vi "实验配置信息读取和写入.vi"(1 "读取写入":bool, 3 "输入簇":T1) -> (9 "输出簇":T1)   [LabVIEW 2010]
uses:
  <vilib>/Utility/config.llb/Read Key (String).vi
  <vilib>/Utility/config.llb/Write Key (String).vi
  <vilib>/Utility/config.llb/NI_LVConfig.lvlib
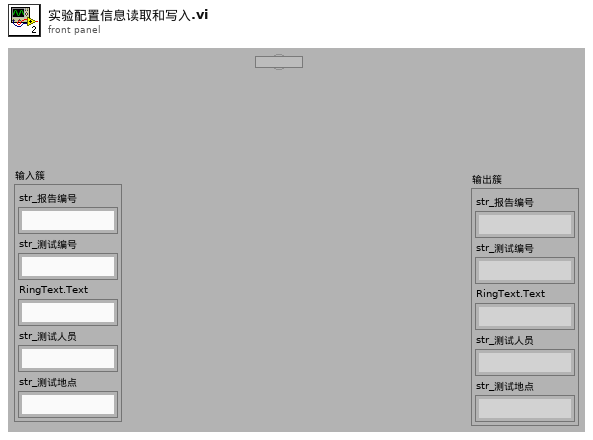
[diagram p1: front panel]
types:
  T1 = cluster{"str_报告编号":string, "str_测试编号":string, "RingText.Text":string, "str_测试人员":string, "str_测试地点":string}
  T2 = typedef "NI_LVConfig.lvlib/Config Data RefNum.ctl" = refnum<k1>
  T3 = cluster{"value":string, "value":string, "value":string, "value":string, "value":string}
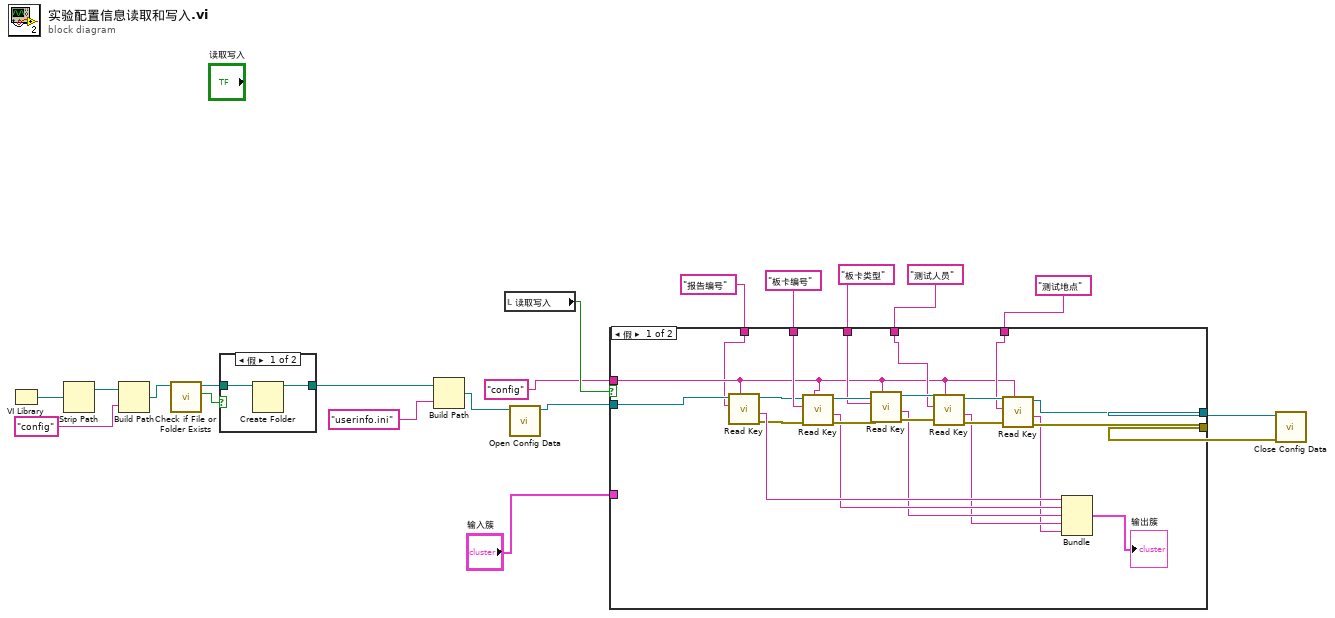
[diagram p0: block diagram]
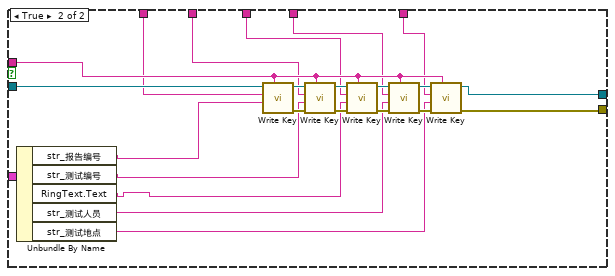
[diagram p2: hidden frame]
diagram:
  n1 = VI Library() -> (path=w19:path)
  n2 = Strip Path(path=w19) -> (stripped path=w20:path)  [unwired: 1 out]
  n3 = Build Path(base path=w20, name or relative path="config") -> (appended path=w17:path)
  n4 = call <vilib>:"Check if File or Folder Exists.vi"("path"=w17) -> ("file or folder exists?"=w16:bool, "dup path"=w15:path)  [unwired: 8 in, 1 out]
  n5 = case shown="假" w16 {
    tunnel: w15 -> [w21 w23]
    tunnel: [w22 w23] -> w14
    frame False {
      n6 = Create Folder(path (use dialog)=w21) -> (created path=w22:path)  [unwired: 2 in, 2 out]
    }
    frame True {
    }
  }
  n7 = Build Path(base path=w14, name or relative path="userinfo.ini" ("名称或相对路径")) -> (appended path=w11:path)
  n8 = local read "读取写入"() -> (w12:bool)
  n9 = call <vilib>:"Open Config Data.vi"("configuration file path"=w11) -> ("refnum"=w9:T2)  [unwired: 8 in, 2 out]
  n10 = case shown="假" w12 {
    tunnel: "config" -> [w32 w61]
    tunnel: w9 -> [w34 w60]
    tunnel: "报告编号" ("key") -> [w31 w59]
    tunnel: "板卡编号" ("key") -> [w43 w58]
    tunnel: "板卡类型" ("key") -> [w42 w57]
    tunnel: "测试人员" ("key") -> [w39 w56]
    tunnel: "测试地点" ("key") -> [w38 w55]
    tunnel: [w41 w54] -> w3
    tunnel: [w40 w53] -> w2
    tunnel: "输入簇" -> [_ w52]
    frame False {
      n11 = call-poly <vilib>:"Read Key.vi"("section"=w32, "key"=w31, "refnum"=w34) -> ("error out"=w29:errorcluster, "value"=w30:string, "refnum out"=w33:T2)  [unwired: 5 in, 1 out]
      n12 = call-poly <vilib>:"Read Key.vi"("section"=w32, "error in (no error)"=w29, "key"=w43, "refnum"=w33) -> ("error out"=w37:errorcluster, "value"=w28:string, "refnum out"=w46:T2)  [unwired: 4 in, 1 out]
      n13 = call-poly <vilib>:"Read Key.vi"("section"=w32, "error in (no error)"=w37, "key"=w42, "refnum"=w46) -> ("error out"=w36:errorcluster, "value"=w27:string, "refnum out"=w45:T2)  [unwired: 4 in, 1 out]
      n14 = call-poly <vilib>:"Read Key.vi"("section"=w32, "error in (no error)"=w36, "key"=w39, "refnum"=w45) -> ("error out"=w35:errorcluster, "value"=w26:string, "refnum out"=w44:T2)  [unwired: 4 in, 1 out]
      n15 = call-poly <vilib>:"Read Key.vi"("section"=w32, "error in (no error)"=w35, "key"=w38, "refnum"=w44) -> ("error out"=w40:errorcluster, "value"=w25:string, "refnum out"=w41:T2)  [unwired: 4 in, 1 out]
      n16 = Bundle("value"=w30, "value"=w28, "value"=w27, "value"=w26, "value"=w25) -> (→"输出簇":T3)  [unwired: 1 in]
    }
    frame True {
      n17 = Unbundle By Name(w52) -> ("str_报告编号"=w51:string, "str_测试编号"=w50:string, "RingText.Text"=w49:string, "str_测试人员"=w48:string, "str_测试地点"=w47:string)
      n18 = call-poly <vilib>:"Write Key.vi"("section"=w61, "value"=w51, "key"=w59, "refnum"=w60) -> ("error out"=w65:errorcluster, "refnum out"=w64:T2)  [unwired: 5 in, 1 out]
      n19 = call-poly <vilib>:"Write Key.vi"("section"=w61, "error in (no error)"=w65, "value"=w50, "key"=w58, "refnum"=w64) -> ("error out"=w67:errorcluster, "refnum out"=w66:T2)  [unwired: 4 in, 1 out]
      n20 = call-poly <vilib>:"Write Key.vi"("section"=w61, "error in (no error)"=w67, "value"=w49, "key"=w57, "refnum"=w66) -> ("error out"=w69:errorcluster, "refnum out"=w68:T2)  [unwired: 4 in, 1 out]
      n21 = call-poly <vilib>:"Write Key.vi"("section"=w61, "error in (no error)"=w69, "value"=w48, "key"=w56, "refnum"=w68) -> ("error out"=w63:errorcluster, "refnum out"=w62:T2)  [unwired: 4 in, 1 out]
      n22 = call-poly <vilib>:"Write Key.vi"("section"=w61, "error in (no error)"=w63, "value"=w47, "key"=w55, "refnum"=w62) -> ("error out"=w53:errorcluster, "refnum out"=w54:T2)  [unwired: 4 in, 1 out]
    }
  }
  n23 = call <vilib>:"Close Config Data.vi"("error in (no error)"=w2, "refnum"=w3) -> ()  [unwired: 8 in, 2 out]
